vi "Handle.vi"(7 "Queue Actor in":refnum<class "Queue Actor.lvclass">, 11 "Error Queue State in":refnum<class "Error Queue State.lvclass">) -> (2 "Destroy?":bool, 5 "Queue Actor out":refnum<class "Queue Actor.lvclass">)   [LabVIEW 2021, in "jettl.lvlib" / "Error Queue State.lvclass"]
uses:
  Error Queue State.lvclass
  Actor/Queue Actor/Queue Actor.lvclass
  Actor/Msgs/Teardown/Teardown Msg/Teardown Msg.lvclass
  C:/git/jettl/src/Actor/Msg/Msg.lvclass
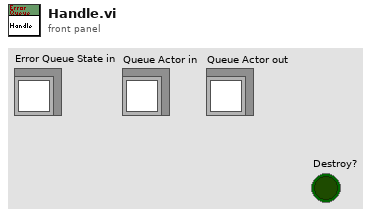
[diagram p1: front panel]
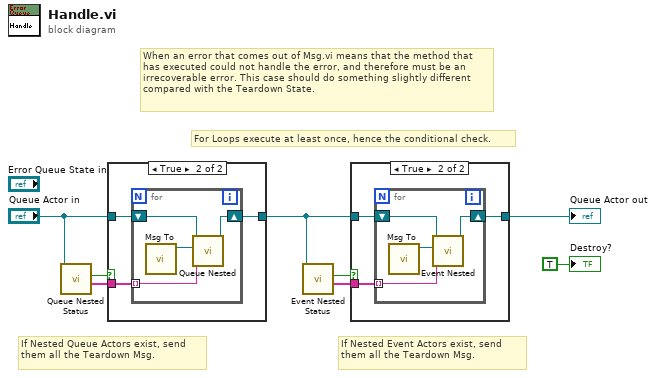
[diagram p0: block diagram]
diagram:
  # "If Nested Event Actors exist, send them all the Teardown Msg."
  # "For Loops execute at least once, hence the conditional check."
  # "If Nested Queue Actors exist, send them all the Teardown Msg."
  # "When an error that comes out of Msg.vi means that the method that has executed could not handle the error, and therefore must be an irrecoverable error. This case should do something slightly different compared with the Teardown State."
  n1 = call-dynamic "Queue Nested Status.vi"("Actor in"="Queue Actor in") -> ("Queue Nested Aliases"=w7:string[], "Any Exist?"=w8:bool)  [unwired: 8 in, 1 out]
  n2 = case shown="True" w8 {
    tunnel: [w9 w12] -> w4
    tunnel: "Queue Actor in" -> [w9 w11]
    tunnel: w7 -> [_ w10]
    frame False {
    }
    frame True {
      n3 = for {
        tunnel: w10 -> [w15] mode=indexing
        shift-right: [w13] -> w12
        shift-left: w11 -> [w14]
        n4 = call "Msg To.vi"() -> ("Teardown Msg out"=w16:refnum<class "Teardown Msg.lvclass">)  [unwired: 11 in]
        n5 = call-dynamic "Queue Nested.vi"("Alias"=w15, "Msg"=w16, "Actor in"=w14) -> ("Actor out"=w13:refnum<class "Queue Actor.lvclass">)  [unwired: 8 in]
      }
    }
  }
  n6 = call-dynamic "Event Nested Status.vi"("Queue Actor in"=w4) -> ("Event Nested Aliases"=w5:string[], "Any Exist?"=w6:bool)  [unwired: 8 in, 1 out]
  n7 = case shown="True" w6 {
    tunnel: [w17 w20] -> w2
    tunnel: w4 -> [w17 w19]
    tunnel: w5 -> [_ w18]
    frame False {
    }
    frame True {
      n8 = for {
        tunnel: w18 -> [w21] mode=indexing
        shift-right: [w23] -> w20
        shift-left: w19 -> [w24]
        n9 = call "Msg To.vi"() -> ("Teardown Msg out"=w22:refnum<class "Teardown Msg.lvclass">)  [unwired: 11 in]
        n10 = call-dynamic "Event Nested.vi"("Alias"=w21, "Msg"=w22, "Queue Actor in"=w24) -> ("Queue Actor out"=w23:refnum<class "Queue Actor.lvclass">)  [unwired: 8 in]
      }
    }
  }
  "Queue Actor out" <- w2
  "Destroy?" <- TRUE ("Destroy?")
